vi "FPGA RoboteQ Driver.vi"(8 "error in (no error)":errorcluster, 9 "FPGA In":T1, 10 "Motor 2 Effort":i32, 11 "Motor 1 Effort":i32) -> (0 "error out":errorcluster, 1 "FPGA Out":T1, 2 "Command to Serial":string, 3 "Byte Count":u32)   [LabVIEW 2012]
uses:
  901x DMA FPGA Reference.ctl
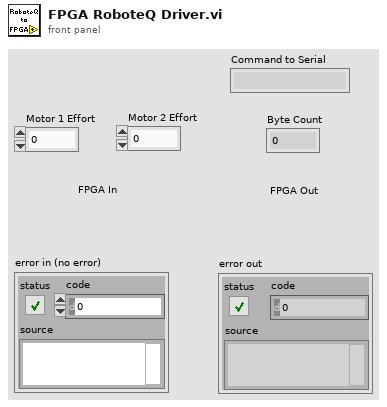
[diagram p1: front panel]
types:
  T1 = typedef "901x DMA FPGA Reference.ctl" = refnum<k20>
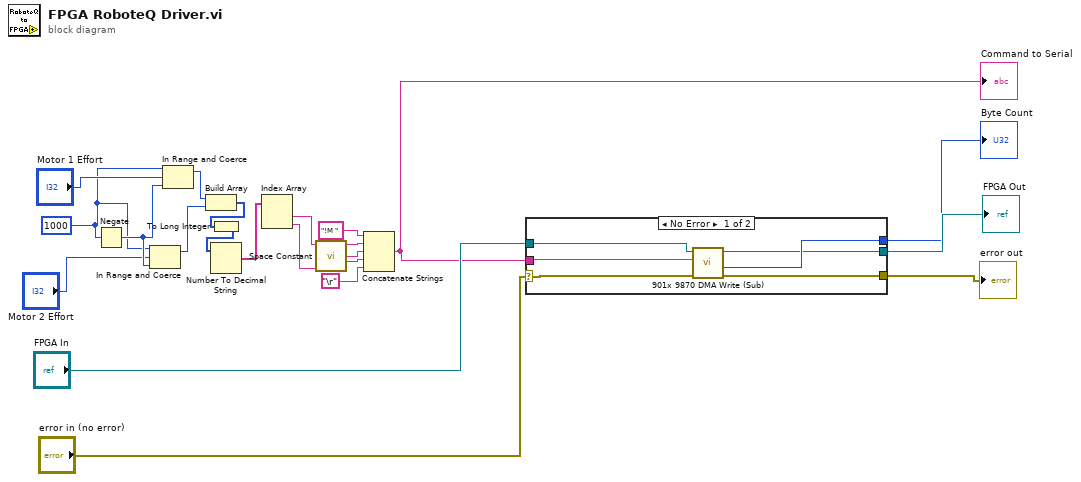
[diagram p0: block diagram]
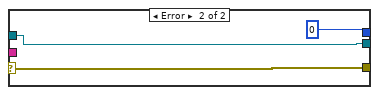
[diagram p2: hidden frame]
diagram:
  w8 = 1000 ("Max Effort")
  n1 = Negate(x=w8) -> (-x=w9:i32)
  n2 = In Range and Coerce(upper limit=w8, x="Motor 2 Effort", lower limit=w9) -> (coerced(x)=w10:i32)  [unwired: 1 out]
  n3 = In Range and Coerce(upper limit=w8, x="Motor 1 Effort", lower limit=w9) -> (coerced(x)=w18:i32)  [unwired: 1 out]
  n4 = Build Array(w18, w10) -> (w17:i32[])
  n5 = To Long Integer(number=w17) -> (32bit integer=w16:i32[])
  n6 = Number To Decimal String(number=w16) -> (decimal integer string=w15:string[])  [unwired: 1 in]
  n7 = Index Array(array=w15) -> (element #1=w13:string, element #2=w12:string)  [unwired: 2 in]
  n8 = call <vilib>:"Space Constant.vi"() -> ("String"=w20:string)
  n9 = Concatenate Strings("!M " ("string"), w13, w20, w12, "\r") -> (w1:string)
  "Command to Serial" <- w1
  n10 = case shown="No Error" "error in (no error)" {
    selector: "error in (no error)" -> [w26 w29]
    tunnel: [w24 w27] -> w3
    tunnel: [w23 w29] -> w5
    tunnel: w1 -> [w22 _]
    tunnel: [w25 0] -> w2
    tunnel: "FPGA In" -> [w21 w27]
    frame No Error {
      n11 = call "901x 9870 DMA Write (Sub).vi"("error in"=w26, "Send Data"=w22, "FPGA In"=w21) -> ("error out"=w23:errorcluster, "Byte Count"=w25:u32, "FPGA Out"=w24:T1)  [unwired: 4 in, 2 out]
    }
    frame Error {
    }
  }
  "error out" <- w5
  "FPGA Out" <- w3
  "Byte Count" <- w2
